vi "Read Control Values from FileProvider_ini.vi"() -> (0 "error out":errorcluster, 1 "Series CFG Path Value":path, 2 "Virt Instrs CFG Value":string, 3 "Virt Instrs CFG Path Value":path, 4 "Series CFG Value":string, 5 "Instrument CFGs":string[](array[string]))   [LabVIEW 2024, in "File Provider.lvlib" / "File Provider.lvclass"]
uses:
  File Provider.lvclass
  File Provider.lvclass/File Provider.ctl
  <vilib>/Utility/config.llb/NI_LVConfig.lvlib
  <vilib>/Utility/config.llb/Read Key (String).vi
  <vilib>/Utility/config.llb/Read Key (Path).vi
  <vilib>/Utility/config.llb/Read Key (I32).vi
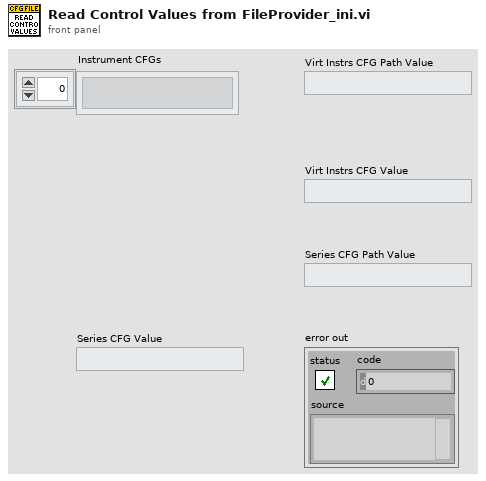
[diagram p1: front panel]
types:
  T1 = typedef "NI_LVConfig.lvlib/Config Data RefNum.ctl" = refnum<k1>
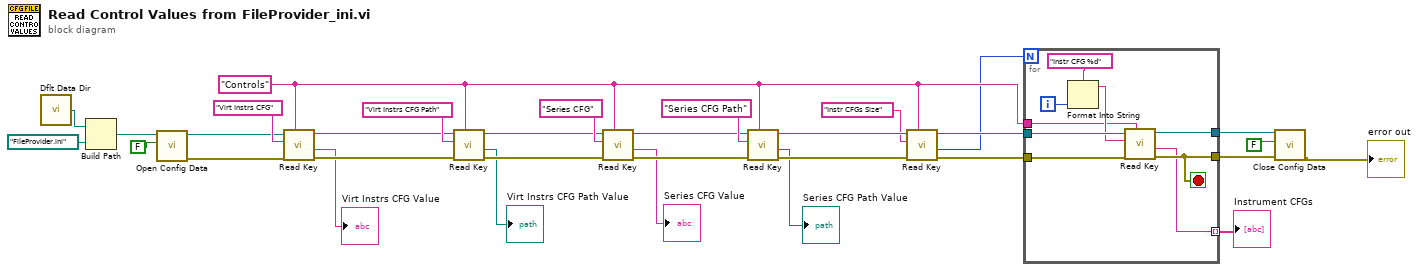
[diagram p0: block diagram]
diagram:
  w2 = "Controls" ("section")
  n1 = call <vilib>:"Dflt Data Dir.vi"() -> ("App:Default Data Directory"=w32:path)
  n2 = Build Path(base path=w32, name or relative path=path "FileProvider.ini" ("default name")) -> (appended path=w14:path)
  n3 = call <vilib>:"Open Config Data.vi"("create file if necessary (T)"=FALSE ("create file if necessary? (T)"), "configuration file path"=w14) -> ("error out"=w20:errorcluster, "refnum"=w19:T1)  [unwired: 1 in, 7 out]
  n4 = call-poly <vilib>:"Read Key.vi"("section"=w2, "error in (no error)"=w20, "key"="Virt Instrs CFG", "refnum"=w19) -> ("error out"=w23:errorcluster, "value"=→"Virt Instrs CFG Value":string, "refnum out"=w28:T1)  [unwired: 4 in, 1 out]
  n5 = call-poly <vilib>:"Read Key.vi"("section"=w2, "error in (no error)"=w23, "key"="Virt Instrs CFG Path", "refnum"=w28) -> ("error out"=w22:errorcluster, "value"=→"Virt Instrs CFG Path Value":path, "refnum out"=w26:T1)  [unwired: 4 in, 1 out]
  n6 = call-poly <vilib>:"Read Key.vi"("section"=w2, "error in (no error)"=w22, "key"="Series CFG", "refnum"=w26) -> ("error out"=w21:errorcluster, "value"=→"Series CFG Value":string, "refnum out"=w24:T1)  [unwired: 4 in, 1 out]
  n7 = call-poly <vilib>:"Read Key.vi"("section"=w2, "error in (no error)"=w21, "key"="Series CFG Path", "refnum"=w24) -> ("error out"=w18:errorcluster, "value"=→"Series CFG Path Value":path, "refnum out"=w5:T1)  [unwired: 4 in, 1 out]
  n8 = call-poly <vilib>:"Read Key.vi"("section"=w2, "error in (no error)"=w18, "key"="Instr CFGs Size" ("format string"), "refnum"=w5) -> ("error out"=w6:errorcluster, "value"=w1:i32, "refnum out"=w4:T1)  [unwired: 4 in, 1 out]
  n9 = for {
    N: w1 -> [_]
    tunnel: w6 -> [w41]
    tunnel: w4 -> [w40]
    tunnel: w2 -> [w36]
    tunnel: [w35] -> w17
    tunnel: [w34] -> w16
    tunnel: [w33] -> w7 mode=indexing
    i -> [w39]
    stop <- w35 stop-if-true
    n10 = Format Into String(format string="Instr CFG %d", w39) -> (resulting string=w37:string)  [unwired: 2 in, 1 out]
    n11 = call-poly <vilib>:"Read Key.vi"("section"=w36, "error in (no error)"=w41, "key"=w37, "refnum"=w40) -> ("error out"=w35:errorcluster, "value"=w33:string, "refnum out"=w34:T1)  [unwired: 4 in, 1 out]
  }
  "Instrument CFGs" <- w7
  n12 = call <vilib>:"Close Config Data.vi"("error in (no error)"=w17, "write file if changed (T)"=FALSE, "refnum"=w16) -> ("error out"=→"error out":errorcluster)  [unwired: 8 out]
